vi "Update Client Control List.vi"(8 "error in (no error)":errorcluster, 10 "Array":string[](array[string]), 11 "Queue in":refnum<queue>) -> (0 "error out":errorcluster, 2 "Command String":string, 3 "Queue out":refnum<queue>)   [LabVIEW 2022 SP3]
doc: "Author: Scott Hannahs <sth@magnet.fsu.edu>\nCopyright 2018 Florida State University, All rights reserved."
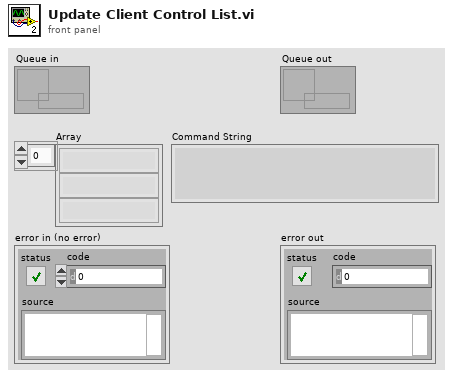
[diagram p1: front panel]
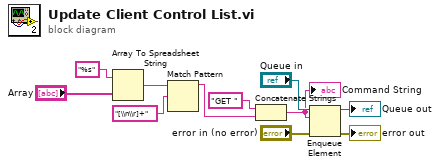
[diagram p0: block diagram]
diagram:
  n1 = Array To Spreadsheet String(array="Array", 3:"%s" ("format string")) -> (spreadsheet string=w3:string)  [unwired: 1 in]
  n2 = Match Pattern(string=w3, regular expression="[\\n\\r]+") -> (before substring=w1:string)  [unwired: 1 in, 3 out]
  n3 = Concatenate Strings("GET " ("string"), w1) -> (w4:string)
  "Command String" <- w4
  n4 = Enqueue Element(queue="Queue in", element=w4, error in (no error)="error in (no error)") -> (queue out=→"Queue out":refnum<queue>, error out=→"error out":errorcluster)  [unwired: 1 in, 1 out]
